vi "Constants.vi"() -> (0 "Constants":T1={"Colours"={"OK"=16777215, "Warning"=16777215, "Error"=16777215, "Red"=16777215, "Green"=16777215, "Blue"=16777215, "Yellow"=16777215, "Health"=16777215, "Energy"=16777215}, "System"={"Target Frames Second"=0.0, "Windows Size"=refnum, "World Size"=refnum, "Battle Area Size"=refnum, "Sidebar Width"=0.0, "SC2 Frame Rate [Seconds/Frame]"=0.0, "Sidebar Player 2 Y Offset"=0.0}, "Game"={"Maximum Asteroids"=0, "Max Energy"=0, "Max Crew"=0, "Maximum Stars"=0}})   [LabVIEW 2021]
uses:
  Re-use Libraries/Vector 2D/Vector 2D.lvclass
  Constants.ctl
  LabSDL2/Source/Libraries/SDL2 Utility/Point (I32).ctl
  LabSDL2/Source/Libraries/SDL2 Utility/SDL2 Utility.lvlib
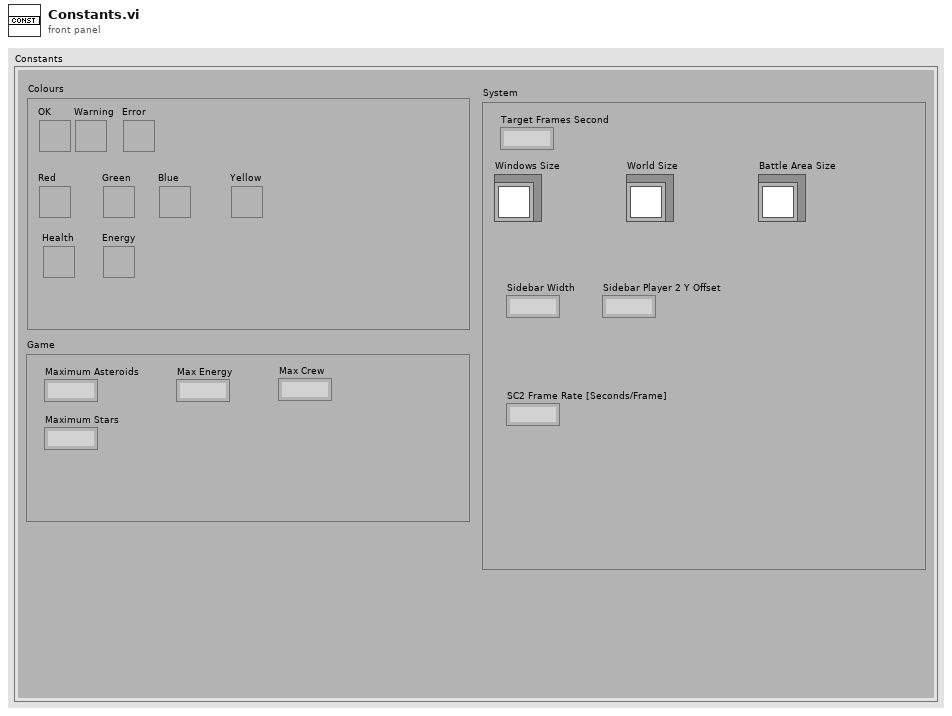
[diagram p1: front panel]
types:
  T1 = typedef "Constants.ctl" = cluster{"Colours":cluster{"OK":u32, "Warning":u32, "Error":u32, "Red":u32, "Green":u32, "Blue":u32, "Yellow":u32, "Health":u32, "Energy":u32}, "System":cluster{"Target Frames Second":dbl, "Windows Size":refnum<class "Vector 2D.lvclass">, "World Size":refnum<class "Vector 2D.lvclass">, "Battle Area Size":refnum<class "Vector 2D.lvclass">, "Sidebar Width":sgl, "SC2 Frame Rate [Seconds/Frame]":sgl, "Sidebar Player 2 Y Offset":sgl}, "Game":cluster{"Maximum Asteroids":i32, "Max Energy":i32, "Max Crew":i32, "Maximum Stars":i32}}
  T2 = typedef "SDL2 Utility.lvlib/Point (I32).ctl" = cluster{"x":i32, "y":i32}
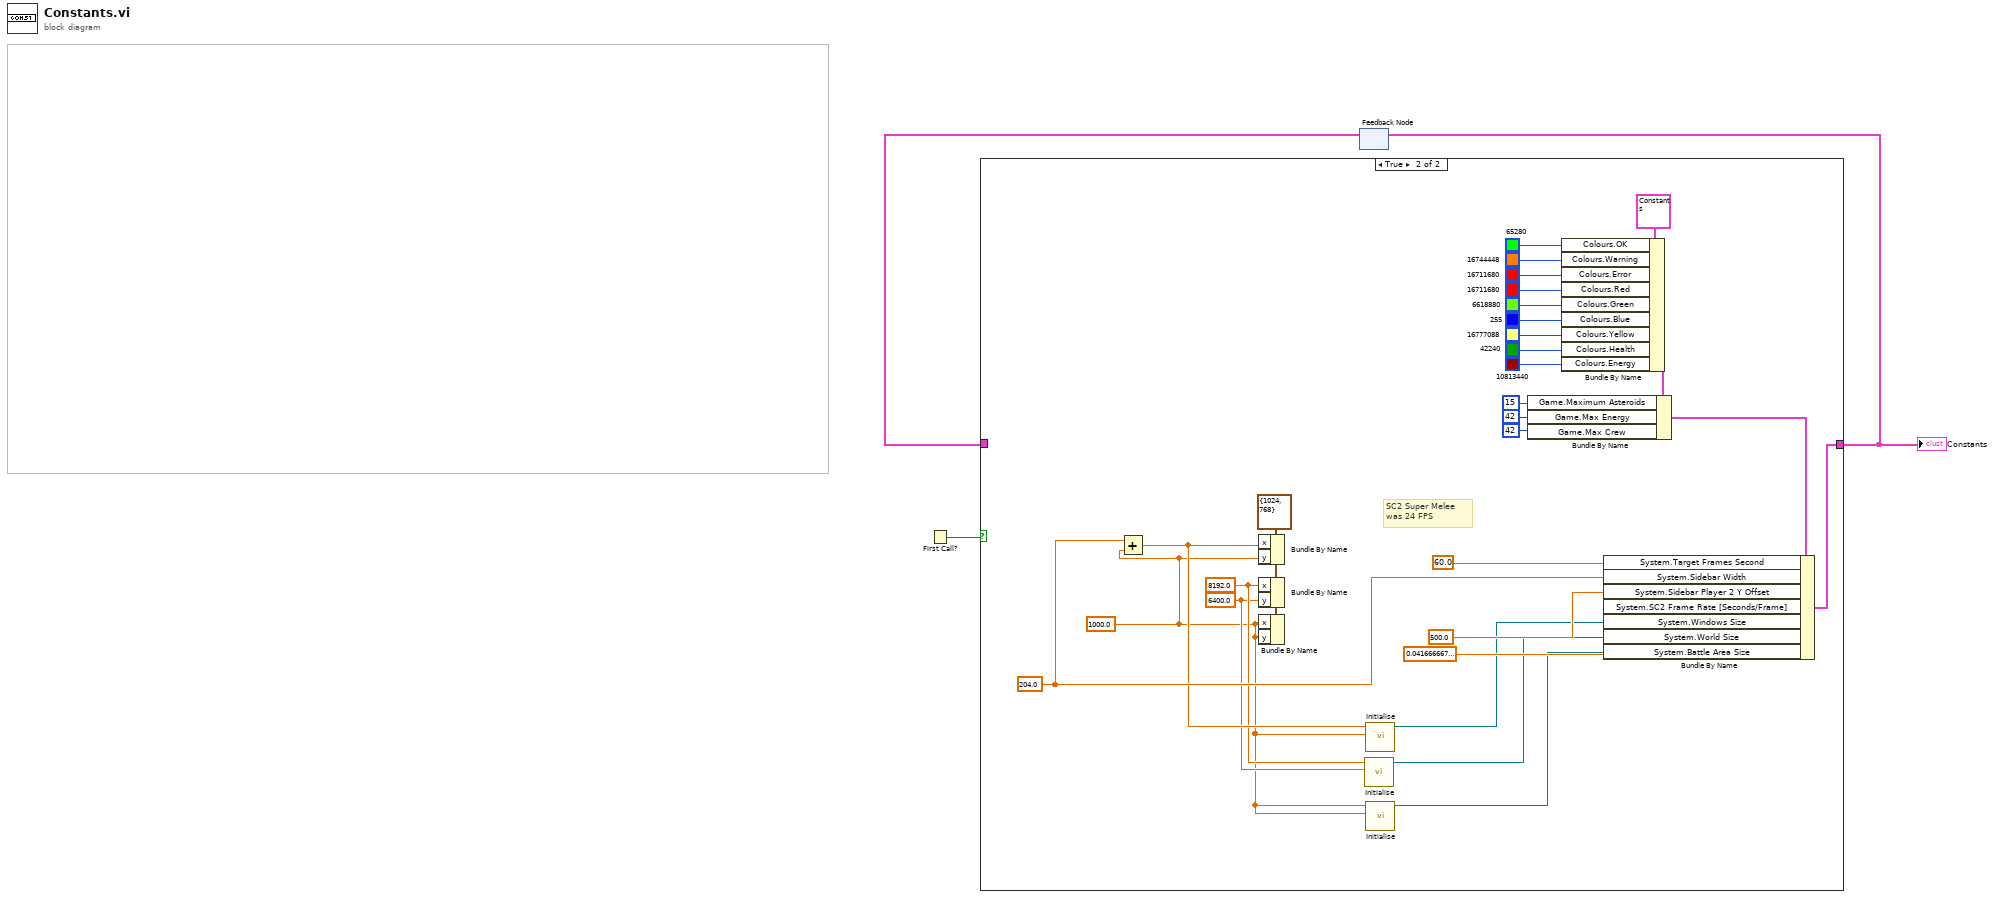
[diagram p0: block diagram]
diagram:
  n1 = First Call?() -> (First Call?: T/F=w3:bool)
  n2 = feedback #1() -> (w1:T1)  [unwired: 1 in]
  n3 = case shown="True" w3 {
    tunnel: [w4 w24] -> w2
    tunnel: w1 -> [w4 _]
    frame False {
    }
    frame True {
      w7 = sgl 1000.0 ("x")
      w8 = sgl 6400.0 ("y")
      w9 = sgl 8192.0 ("x")
      w23 = T2 {"x"=1024, "y"=768} ("System.Field Size")
      w18 = sgl 204.0 ("System.Sidebar Width")
      # "SC2 Super Melee was 24 FPS"
      n4 = Add(x=w18, y=w7) -> (x+y=w12:sgl)
      n5 = Bundle By Name(cluster=w23, "x"=w12, "y"=w7) -> ()  [unwired: 1 out]
      n6 = Bundle By Name(cluster=w23, "x"=w9, "y"=w8) -> ()  [unwired: 1 out]
      n7 = Bundle By Name(cluster=w23, "x"=w7, "y"=w7) -> ()  [unwired: 1 out]
      n8 = call "Initialise.vi"("y"=w8, "x"=w9) -> ("Vector 2D out"=w11:refnum<class "Vector 2D.lvclass">)  [unwired: 9 in]
      n9 = call "Initialise.vi"("y"=w7, "x"=w12) -> ("Vector 2D out"=w13:refnum<class "Vector 2D.lvclass">)  [unwired: 9 in]
      n10 = call "Initialise.vi"("y"=w7, "x"=w7) -> ("Vector 2D out"=w10:refnum<class "Vector 2D.lvclass">)  [unwired: 9 in]
      n11 = Bundle By Name(cluster=T1 {"Colours"={"OK"=16777215, "Warning"=16777215, "Error"=16777215, "Red"=16777215, "Green"=16777215, "Blue"=16777215, "Yellow"=16777215, "Health"=16777215, "Energy"=16777215}, "System"={"Target Frames Second"=0.0, "Windows Size"=refnum, "World Size"=refnum, "Battle Area Size"=refnum, "Sidebar Width"=0.0, "SC2 Frame Rate [Seconds/Frame]"=0.0, "Sidebar Player 2 Y Offset"=0.0}, "Game"={"Maximum Asteroids"=0, "Max Energy"=0, "Max Crew"=0, "Maximum Stars"=0}} ("Constants"), "Colours.OK"=u32 65280 ("Colour - OK"), "Colours.Warning"=u32 16744448 ("Colour - Warning"), "Colours.Error"=u32 16711680 ("Colour - Error"), "Colours.Red"=u32 16711680 ("Colour - OK"), "Colours.Green"=u32 6618880 ("Colour - Warning"), "Colours.Blue"=u32 255 ("Colour - Error"), "Colours.Yellow"=u32 16777088 ("Colour - OK"), "Colours.Health"=u32 42240 ("Colour - OK"), "Colours.Energy"=u32 10813440 ("Colour - OK")) -> (w27:T1)
      n12 = Bundle By Name(cluster=w27, "Game.Maximum Asteroids"=15, "Game.Max Energy"=42, "Game.Max Crew"=42) -> (w26:T1)
      n13 = Bundle By Name(cluster=w26, "System.Target Frames Second"=60.0 ("Misc.Number Of Stations"), "System.Sidebar Width"=w18, "System.Sidebar Player 2 Y Offset"=sgl 500.0, "System.SC2 Frame Rate [Seconds/Frame]"=sgl 0.041666668 ("1/x"), "System.Windows Size"=w13, "System.World Size"=w11, "System.Battle Area Size"=w10) -> (w24:T1)
    }
  }
  "Constants" <- w2
  n14 = feedback-in #1(w2) -> ()
